vi "Get First VI Call Chain with Open Panel.vi"(8 "error in (no error)":errorcluster) -> (0 "error out":errorcluster, 2 "Panel Found":bool, 3 "vi reference":refnum<vi>)   [LabVIEW 2023]
doc: "Work up the call chain form this VI's calling VI and return a reference to the first VI with an open front panel.\n\nThis is required for defer panel updates or other methods which require an open front panel."
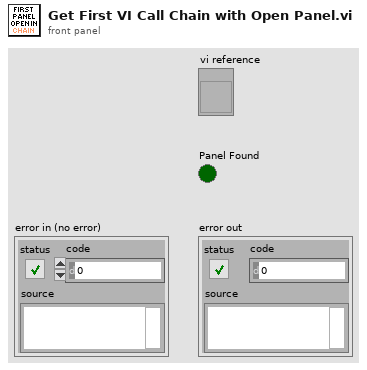
[diagram p1: front panel]
types:
  T1 = enum32{"Invalid", "Standard", "Closed", "Hidden", "Minimized", "Maximized"}
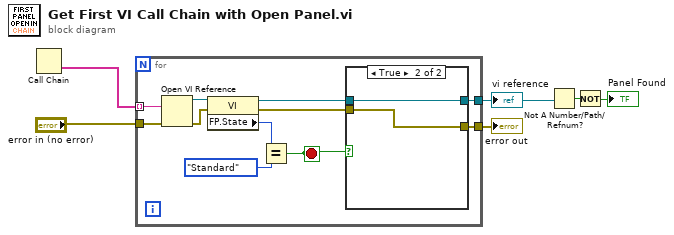
[diagram p0: block diagram]
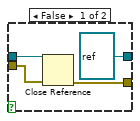
[diagram p2: hidden frame]
diagram:
  n1 = Call Chain() -> (call chain=w4:string[])
  n2 = for {
    tunnel: w4 -> [w17] mode=indexing
    tunnel: [w11] -> w3
    tunnel: "error in (no error)" -> [w10]
    tunnel: [w7] -> w6
    stop <- w12 stop-if-true
    n3 = Open VI Reference(vi path=w17, error in (no error)=w10) -> (vi reference=w16:refnum<vi>, error out=w9:errorcluster)  [unwired: 4 in]
    n4 = property class="VI"(reference=w16, error in=w9) -> (reference out=w13:refnum<vi>, error out=w8:errorcluster, "FP.State"=w14:T1)
    n5 = Equal?(x=w14, y=T1."Standard" ("Front Panel Window:State")) -> (x = y?=w12:bool)
    n6 = case shown="True" w12 {
      tunnel: w13 -> [w21 w23]
      tunnel: [refnum<vi> refnum ("vi reference") w23] -> w11
      tunnel: w8 -> [w19 w22]
      tunnel: [w18 w22] -> w7
      frame False {
        n7 = Close Reference(reference=w21, error in (no error)=w19) -> (error out=w18:errorcluster)
      }
      frame True {
      }
    }
  }
  "error out" <- w6
  "vi reference" <- w3
  n8 = Not A Number/Path/Refnum?(number/path/refnum=w3) -> (NaN/Path/Refnum?=w2:bool)
  n9 = Not(x=w2) -> (.not. x?=→"Panel Found":bool)
